vi "ge_WhichClassSelected.vi"(8 "error in":errorcluster, 10 "LS Chan Groups":refnum<vi>, 11 "HS Chan Groups":refnum<vi>) -> (0 "error out":errorcluster, 2 "Selected Group":T1)   [LabVIEW 2011]
uses:
  Custom Ctrls/ge_SelectedGroup.ctl
  Custom Ctrls/ge_TimingEngine.ctl
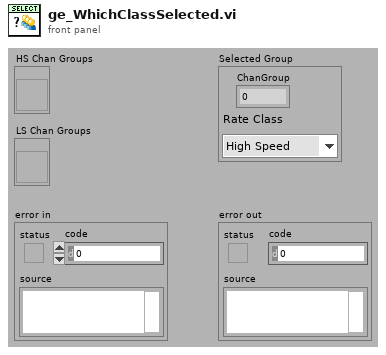
[diagram p1: front panel]
types:
  T1 = typedef "ge_SelectedGroup.ctl" = cluster{"ChanGroup":i32, "Rate Class":T2}
  T2 = typedef "ge_TimingEngine.ctl" = enum16{"High Speed", "Low Speed"}
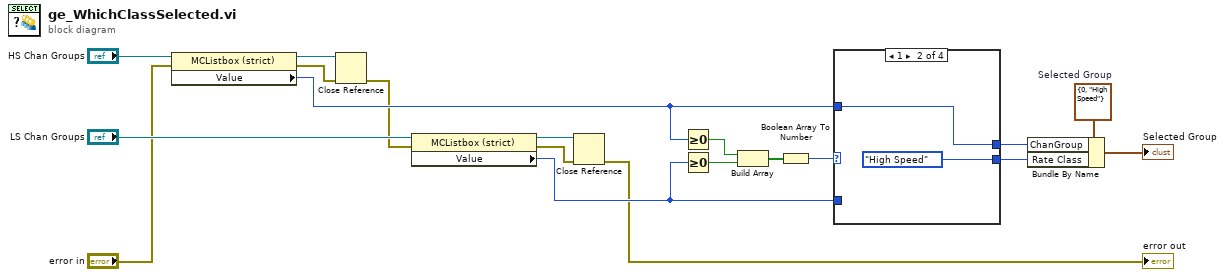
[diagram p0: block diagram]
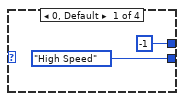
[diagram p2: hidden frame]
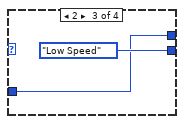
[diagram p3: hidden frame]
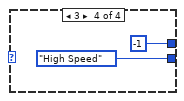
[diagram p4: hidden frame]
diagram:
  w15 = T1 {"ChanGroup"=0, "Rate Class"=enum."High Speed"}  # Selected Group
  n1 = property on="Property Node" class="MCListbox (strict)"(reference="HS Chan Groups", error in="error in") -> (reference out=w11:refnum<vi>, error out=w9:errorcluster, "Value"=w5:i32)
  n2 = Close Reference(reference=w11, error in (no error)=w9) -> (error out=w3:errorcluster)
  n3 = property on="Property Node" class="MCListbox (strict)"(reference="LS Chan Groups", error in=w3) -> (reference out=w7:refnum<vi>, error out=w8:errorcluster, "Value"=w4:i32)
  n4 = Close Reference(reference=w7, error in (no error)=w8) -> (error out=→"error out":errorcluster)
  n5 = Greater Or Equal To 0?(x=w5) -> (x >= 0?=w18:bool)
  n6 = Greater Or Equal To 0?(x=w4) -> (x >= 0?=w19:bool)
  n7 = Build Array(w18, w19) -> (w17:bool[])
  n8 = Boolean Array To Number(Boolean array=w17) -> (number=w16:u32)
  n9 = case shown="1" w16 {
    tunnel: [ge_TimingEngine."High Speed" ("Rate Class") ge_TimingEngine."High Speed" ("Rate Class") ge_TimingEngine."Low Speed" ("Rate Class") ge_TimingEngine."High Speed" ("Rate Class")] -> w13
    tunnel: w5 -> [_ w22 _ _]
    tunnel: w4 -> [_ _ w24 _]
    tunnel: [-1 ("LS Chan Groups") w22 w24 -1 ("LS Chan Groups")] -> w14
    frame 0, Default {
    }
    frame 1 {
    }
    frame 2 {
    }
    frame 3 {
    }
  }
  n10 = Bundle By Name(cluster=w15, "ChanGroup"=w14, "Rate Class"=w13) -> (→"Selected Group":T1)
